vi "ReceptionRS232.vi"(0 "VISA in":refnum<visa-resource-name>, 1 "Erreur in":errorcluster) -> (2 "VISA out":refnum<visa-resource-name>, 3 "Réponse":string, 4 "Erreur out":errorcluster)   [LabVIEW 2011]
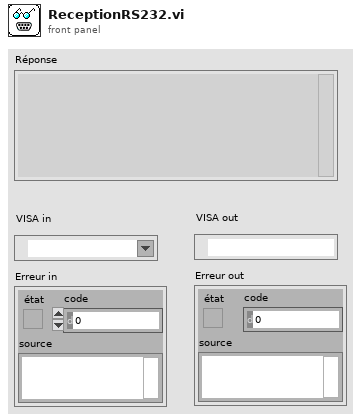
[diagram p1: front panel]
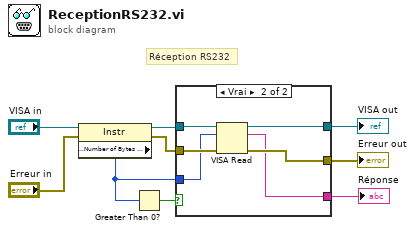
[diagram p0: block diagram]
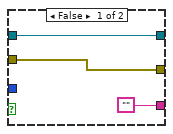
[diagram p2: hidden frame]
diagram:
  # "Réception RS232"
  n1 = property class="Instr"(reference="VISA in", error in="Erreur in") -> (reference out=w6:refnum<visa-resource-name>, error out=w7:errorcluster, "Serial Settings:Number of Bytes at Serial Port"=w8:u32)
  n2 = Greater Than 0?(x=w8) -> (x > 0?=w9:bool)
  n3 = case shown="Vrai" w9 {
    tunnel: w6 -> [w12 w18]
    tunnel: [w12 w17] -> w4
    tunnel: w7 -> [w11 w16]
    tunnel: [w11 w15] -> w3
    tunnel: ["" w13] -> w5
    tunnel: w8 -> [_ w14]
    frame False {
    }
    frame True {
      n4 = VISA Read(VISA resource name=w18, byte count=w14, error in (no error)=w16) -> (VISA resource name out=w17:refnum<visa-resource-name>, read buffer=w13:string, error out=w15:errorcluster)  [unwired: 1 out]
    }
  }
  "VISA out" <- w4
  "Erreur out" <- w3
  "Réponse" <- w5
